vi "GetSize.vi"(8 "Error In":errorcluster, 11 "object in":refnum<class "Board Game.lvclass">) -> (0 "Error Out":errorcluster, 2 "Size":u16, 3 "object out":refnum<class "Board Game.lvclass">)   [LabVIEW 2021, in "Board Game.lvclass"]
uses:
  Board Game.lvclass
  Board Game.lvclass/Board Game.ctl
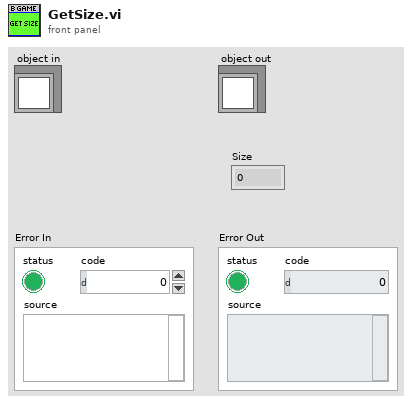
[diagram p1: front panel]
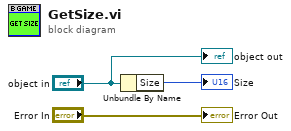
[diagram p0: block diagram]
diagram:
  n1 = Unbundle By Name("object in") -> ("Size"=→"Size":u16)
  "Error Out" <- "Error In"
  "object out" <- "object in"
